vi "DataInFPYALRev.1.0.vi"(9 "P/F":string, 10 "SN":string, 11 "FixtureName":string) -> ()   [LabVIEW 2011]
panel:
  out "Ctrl+V":string
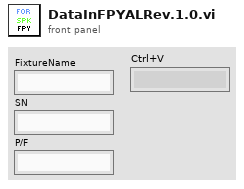
[diagram p1: front panel]
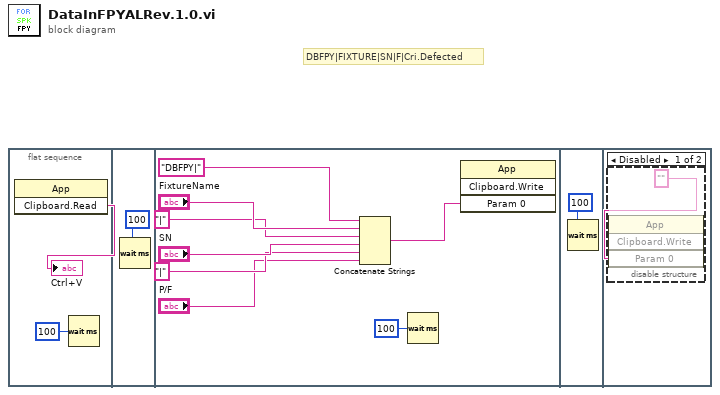
[diagram p0: block diagram]
diagram:
  # "DBFPY|FIXTURE|SN|F|Cri.Defected"
  n1 = flat-sequence {
    frame #0 {
      n2 = invoke class="App" method="Clipboard.Read"() -> ("Read Clipbrd"=→"Ctrl+V":string)  [unwired: 3 in, 2 out]
      n3 = Wait (ms)(milliseconds to wait=u32 100) -> ()  [unwired: 1 out]
    }
    frame #1 {
      n4 = Wait (ms)(milliseconds to wait=u32 100) -> ()  [unwired: 1 out]
    }
    frame #2 {
      n5 = Concatenate Strings("DBFPY|", "FixtureName", "|" ("string"), "SN", "|" ("string"), "P/F") -> (w5:string)
      n6 = Wait (ms)(milliseconds to wait=u32 100) -> ()  [unwired: 1 out]
      n7 = invoke class="App" method="Clipboard.Write"("Param 0"=w5) -> ()  [unwired: 3 in, 4 out]
    }
    frame #3 {
      n8 = Wait (ms)(milliseconds to wait=u32 100) -> ()  [unwired: 1 out]
    }
    frame #4 {
      n9 = disable-structure shown="Disabled" {
        frame Disabled {
          n10 = invoke class="App" method="Clipboard.Write"("Param 0"="") -> ()  [unwired: 3 in, 4 out]
        }
        frame Enabled {
        }
      }
    }
  }
